vi "SendAutotestResult.vi"(8 "error in (no error)":errorcluster, 11 "Message":T1) -> (0 "error out":errorcluster)   [LabVIEW 2011]
uses:
  030 - EVENTS/03 - ToMessageHandlerProcess/ToMessageHandlerEvent.ctl
  030 - EVENTS/03 - ToMessageHandlerProcess/enumMessageCriticity.ctl
  030 - EVENTS/EnumFgvEventCommand.ctl
  030 - EVENTS/05 - FromProcesses/FromProcessEvent.ctl
  030 - EVENTS/05 - FromProcesses/FromProcessesEventType.ctl
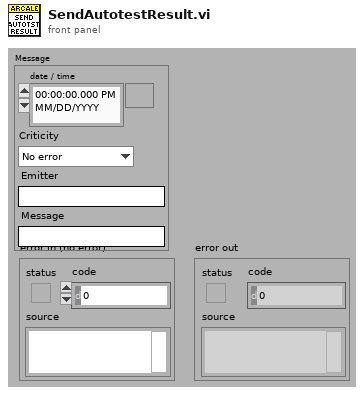
[diagram p1: front panel]
types:
  T1 = typedef "ToMessageHandlerEvent.ctl" = cluster{"date / time":timestamp, "Criticity":T2, "Emitter":string, "Message":string}
  T2 = typedef "enumMessageCriticity.ctl" = enum16{"No error", "Info", "Warning", "Error", "Fatal error"}
  T3 = typedef "FromProcessesEventType.ctl" = enum16{"Started", "Autotest", "Ended"}
  T4 = typedef "FromProcessEvent.ctl" = cluster{"Command":T3, "Process path":path, "Message":T1, "Process Refnum":refnum<vi>}
  T5 = typedef "EnumFgvEventCommand.ctl" = enum16{"Setup", "Cleanup", "Get"}
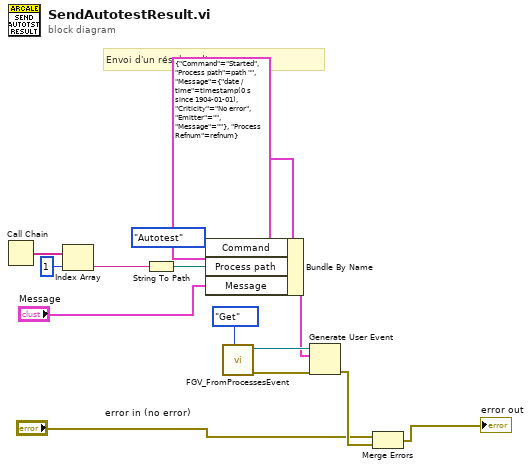
[diagram p0: block diagram]
diagram:
  # "Envoi d'un résultat d'autotest ..."
  n1 = Call Chain() -> (call chain=w5:string[])
  n2 = Index Array(array=w5, index=1) -> (element=w3:string)
  n3 = String To Path(string=w3) -> (path=w2:path)
  n4 = Bundle By Name(cluster=T4 {"Command"=enum."Started", "Process path"=path "", "Message"={"date / time"=timestamp(0 s since 1904-01-01), "Criticity"=enum."No error", "Emitter"="", "Message"=""}, "Process Refnum"=refnum} ("event data"), "Command"=FromProcessesEventType."Autotest", "Process path"=w2, "Message"="Message") -> (w7:T4)
  n5 = call "FGV_FromProcessesEvent.vi"("Command"=EnumFgvEventCommand."Get") -> ("error out"=w13:errorcluster, "From Process Event"=w12:refnum<user-event>)  [unwired: 9 in]
  n6 = Generate User Event(user event=w12, event data cluster=w7, error in=w13) -> (error out=w11:errorcluster)  [unwired: 1 out]
  n7 = Merge Errors("error in (no error)", w11) -> (→"error out":errorcluster)
